vi "Read Slope.vi"(8 "error in (no error)":errorcluster, 11 "Frequency in":refnum<class "Frequency.lvclass">) -> (0 "error out":errorcluster, 2 "Slope":u16, 3 "Frequency out":refnum<class "Frequency.lvclass">)   [LabVIEW 2018, in "Measurement Channels.lvlib" / "Frequency.lvclass"]
uses:
  Frequency.lvclass
  Frequency.lvclass/Frequency.ctl
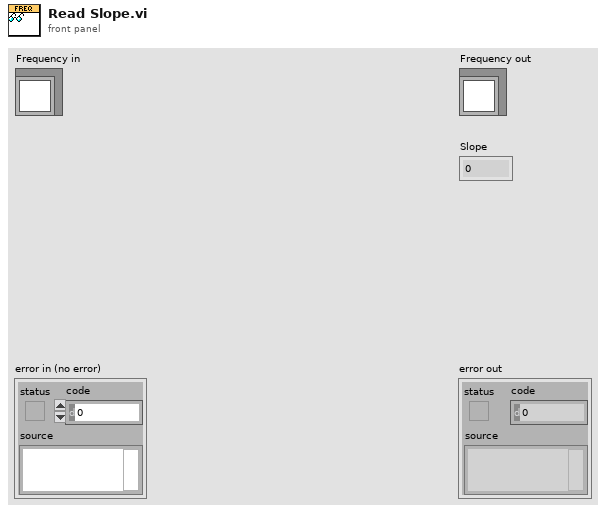
[diagram p1: front panel]
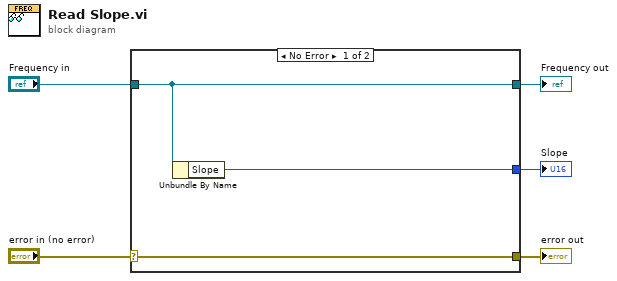
[diagram p0: block diagram]
diagram:
  n1 = case shown="No Error" "error in (no error)" {
    selector: "error in (no error)" -> [w8 w9]
    tunnel: [w8 w9] -> w4
    tunnel: [w7 w10] -> w2
    tunnel: "Frequency in" -> [w7 w10]
    tunnel: [w6 _] -> w1
    frame No Error {
      n2 = Unbundle By Name(w7) -> ("Slope"=w6:u16)
    }
    frame Error {
    }
  }
  "error out" <- w4
  "Frequency out" <- w2
  "Slope" <- w1
